vi "AutoApproach_rawspeed.vi"() -> ()   [LabVIEW 2019]
doc: "Programming Interface Example: Automatic approach implemented using Nanonis Programming Interface functions. This can be used if you want to execute special functions after each motor step or if you want to control your motor directly from LabVIEW.\n\n- Nanonis Programming Interface -"
uses:
  GlobalClicksHeight_raw.vi
  <userlib>/Nanonis Prog Interface V5/Nanonis Prog Interface.lvlib
panel:
  in  "Motor steps":u16=1
  in  "Wait for motor (ms)":u32=1000
  in  "stop":bool
  out "Surface reached":bool
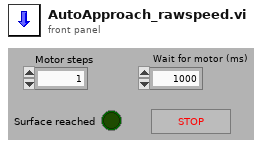
[diagram p1: front panel]
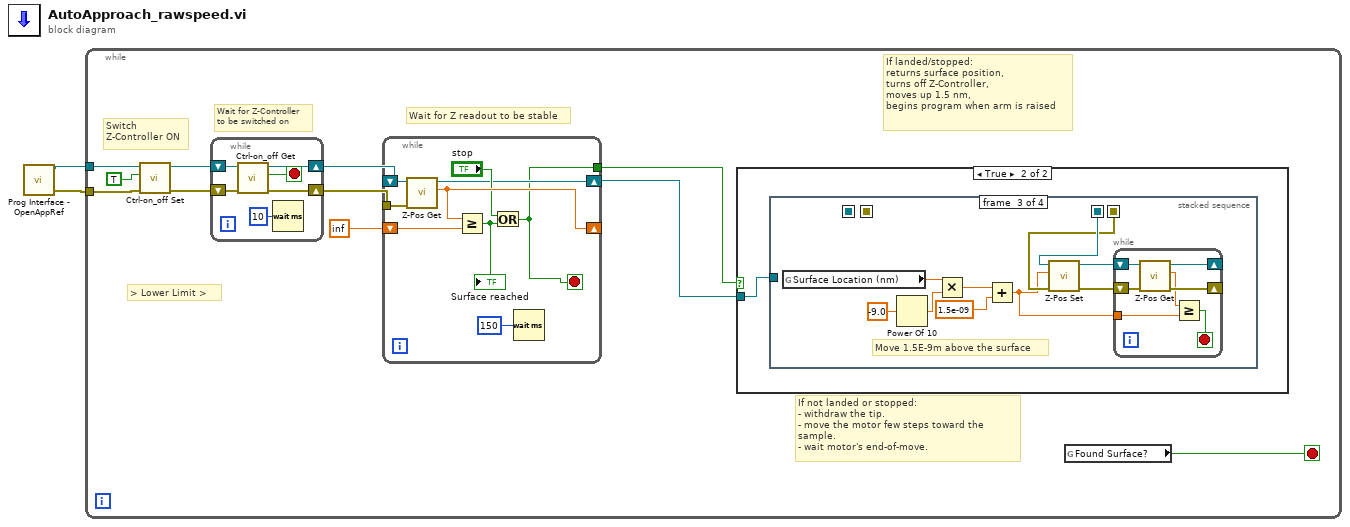
[diagram p0: block diagram]
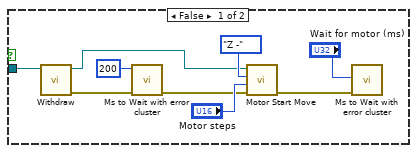
[diagram p2: hidden frame]
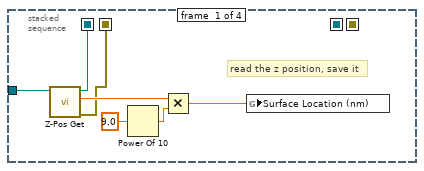
[diagram p3: hidden frame]
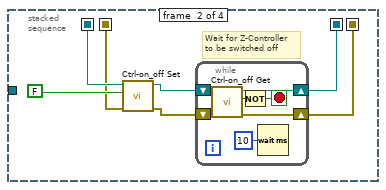
[diagram p4: hidden frame]
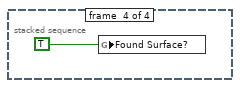
[diagram p5: hidden frame]
diagram:
  n1 = call <userlib>:"Prog Interface - OpenAppRef.vi"() -> ("Error out"=w1:errorcluster, "Application reference"=w2:refnum<vi>)  [unwired: 6 in]
  n2 = while {
    tunnel: w2 -> [w4]
    tunnel: w1 -> [w3]
    stop <- w5 stop-if-true
    # "Wait for Z readout to be stable"
    # "If landed/stopped:  \nreturns surface position, \nturns off Z-Controller, \nmoves up 1.5 nm,\nbegins program when arm is raised"
    # "Wait for Z-Controller\nto be switched on"
    # "> Lower Limit >"
    # "Switch Z-Controller ON"
    # "If not landed or stopped:\n- withdraw the tip.\n- move the motor few steps toward the sample.\n- wait motor's end-of-move."
    n3 = call <userlib>:"Ctrl-on_off Set.vi"("error in (no error)"=w3, "Z Controller ON/OFF"=TRUE ("Ctrl on/off"), "Application ref in"=w4) -> ("error out"=w10:errorcluster, "Application ref out"=w8:refnum<vi>)  [unwired: 7 in]
    n4 = while {
      shift-right: [w19] -> w9
      shift-left: w10 -> [w18]
      shift-right: [w14] -> w7
      shift-left: w8 -> [w15]
      stop <- w17 stop-if-true
      n5 = call <userlib>:"Ctrl-on_off Get.vi"("error in (no error)"=w18, "Application ref in"=w15) -> ("error out"=w19:errorcluster, "Z-Controller on/off status"=w17:bool, "Application ref out"=w14:refnum<vi>)  [unwired: 7 in]
      n6 = Wait (ms)(milliseconds to wait=u32 10) -> ()  [unwired: 1 out]
    }
    n7 = while {
      shift-right: [w26] -> _
      shift-left: sgl inf ("Z-pos (m)") -> [w28]
      tunnel: [w20] -> w13
      tunnel: w9 -> [w23]
      shift-right: [w21] -> w6
      shift-left: w7 -> [w22]
      stop <- w20 stop-if-true
      n8 = call <userlib>:"Z-Pos Get.vi"("error in (no error)"=w23, "Application ref in"=w22) -> ("Z position (m)"=w26:sgl, "Application ref out"=w21:refnum<vi>)  [unwired: 7 in, 1 out]
      n9 = Greater Or Equal?(x=w26, y=w28) -> (x >= y?=w25:bool)
      "Surface reached" <- w25
      n10 = Or(x="stop", y=w25) -> (x .or. y?=w20:bool)
      n11 = Wait (ms)(milliseconds to wait=u32 150) -> ()  [unwired: 1 out]
    }
    n12 = case shown="True" w13 {
      tunnel: w6 -> [w30 w38]
      frame False {
        n13 = call <userlib>:"Withdraw.vi"("Application ref in"=w30) -> ("Error out"=w35:errorcluster, "Application ref out"=w29:refnum<vi>)  [unwired: 9 in]
        n14 = call <userlib>:"Ms to Wait with error cluster.vi"("error in (no error)"=w35, "milliseconds to wait"=u32 200) -> ("error out"=w34:errorcluster)  [unwired: 4 in, 1 out]
        n15 = call <userlib>:"Motor Start Move.vi"("Error in (no error)"=w34, "Number of steps"="Motor steps", "Direction"=enum16{"X +", "X -", "Y +", "Y -", "Z +", "Z -"}."Z -", "Application ref in"=w29) -> ("Error out"=w32:errorcluster)  [unwired: 5 in, 1 out]
        n16 = call <userlib>:"Ms to Wait with error cluster.vi"("error in (no error)"=w32, "milliseconds to wait"="Wait for motor (ms)") -> ()  [unwired: 4 in, 2 out]
      }
      frame True {
        n17 = stacked-sequence {
          seq-local: [w42 _ _ _] -> [_ w51 _ _]
          seq-local: [w40 _ _ _] -> [_ w50 _ _]
          seq-local: [_ w47 _ _] -> [_ _ w65 _]
          seq-local: [_ w46 _ _] -> [_ _ w64 _]
          tunnel: w38 -> [w41 _ _ _]
          frame #0 {
            # "read the z position, save it"
            n18 = call <userlib>:"Z-Pos Get.vi"("Application ref in"=w41) -> ("error out"=w40:errorcluster, "Z position (m)"=w45:sgl, "Application ref out"=w42:refnum<vi>)  [unwired: 8 in]
            n19 = Power Of 10(x=9.0) -> (10^x=w44:dbl)
            n20 = Multiply(x=w45, y=w44) -> (x*y=w39:dbl)
            n21 = global write "GlobalClicksHeight_raw.vi" "Surface Location (nm)"(w39) -> ()
          }
          frame #1 {
            # "Wait for Z-Controller\nto be switched off"
            n22 = call <userlib>:"Ctrl-on_off Set.vi"("error in (no error)"=w50, "Z Controller ON/OFF"=FALSE, "Application ref in"=w51) -> ("error out"=w48:errorcluster, "Application ref out"=w49:refnum<vi>)  [unwired: 7 in]
            n23 = while {
              shift-right: [w59] -> w46
              shift-left: w48 -> [w58]
              shift-right: [w54] -> w47
              shift-left: w49 -> [w55]
              stop <- w53 stop-if-true
              n24 = call <userlib>:"Ctrl-on_off Get.vi"("error in (no error)"=w58, "Application ref in"=w55) -> ("error out"=w59:errorcluster, "Z-Controller on/off status"=w57:bool, "Application ref out"=w54:refnum<vi>)  [unwired: 7 in]
              n25 = Not(x=w57) -> (.not. x?=w53:bool)
              n26 = Wait (ms)(milliseconds to wait=u32 10) -> ()  [unwired: 1 out]
            }
          }
          frame #2 {
            # "Move 1.5E-9m above the surface"
            n27 = global read "GlobalClicksHeight_raw.vi" "Surface Location (nm)"() -> (w60:dbl)
            n28 = Power Of 10(x=-9.0) -> (10^x=w69:dbl)
            n29 = Multiply(x=w60, y=w69) -> (x*y=w67:dbl)
            n30 = Add(x=w67, y=1.5e-09) -> (x+y=w61:dbl)
            n31 = call <userlib>:"Z-Pos Set.vi"("error in (no error)"=w64, "Z position (m)"=w61, "Application ref in"=w65) -> ("error out"=w62:errorcluster, "Application ref out"=w63:refnum<vi>)  [unwired: 7 in]
            n32 = while {
              shift-right: [w73] -> _
              shift-left: w62 -> [w75]
              shift-right: [w74] -> _
              shift-left: w63 -> [w76]
              tunnel: w61 -> [w70]
              stop <- w72 stop-if-true
              n33 = call <userlib>:"Z-Pos Get.vi"("error in (no error)"=w75, "Application ref in"=w76) -> ("error out"=w73:errorcluster, "Z position (m)"=w71:sgl, "Application ref out"=w74:refnum<vi>)  [unwired: 7 in]
              n34 = Greater Or Equal?(x=w71, y=w70) -> (x >= y?=w72:bool)
            }
          }
          frame #3 {
            n35 = global write "GlobalClicksHeight_raw.vi" "Found Surface?"(TRUE ("Clicks and Height")) -> ()
          }
        }
      }
    }
    n36 = global read "GlobalClicksHeight_raw.vi" "Found Surface?"() -> (w5:bool)
  }
